vi "Page_Info_Read.vi"(6 "ctlReferences":T1, 8 "error in (no error)":errorcluster, 11 "AB_Deploy_EXE in":refnum<class "AB_Deploy_EXE.lvclass">) -> (0 "error out":errorcluster, 3 "AB_Deploy_EXE out":refnum<class "AB_Deploy_EXE.lvclass">)   [LabVIEW 2020, in "AB_Deploy_EXE.lvclass"]
uses:
  <vilib>/AppBuilder/AB_Classes/DeployableEXE/AB_Deploy_EXE.lvclass
  e:/builds/penguin/labview/branches/2020/dev/dist/vi.lib/AppBuilder/AB_Classes/Build/AB_Build.lvclass
  e:/builds/penguin/labview/branches/2020/dev/dist/vi.lib/AppBuilder/AB_Classes/TargetFile/AB_Targetfile.lvclass
  <resource>/Framework/Providers/Builds/AppBuilder/AB_UI_Page_Info_References.ctl
  <vilib>/AppBuilder/AB_Classes/DeployableEXE/AB_Deploy_EXE.lvclass/AB_Deploy_EXE.ctl
  <vilib>/AppBuilder/AB_Classes/Destination/AB_Destination.lvclass
  <vilib>/AppBuilder/AB_Classes/Build/AB_Build.lvclass
  <vilib>/AppBuilder/AB_Classes/TargetFile/AB_Targetfile.lvclass
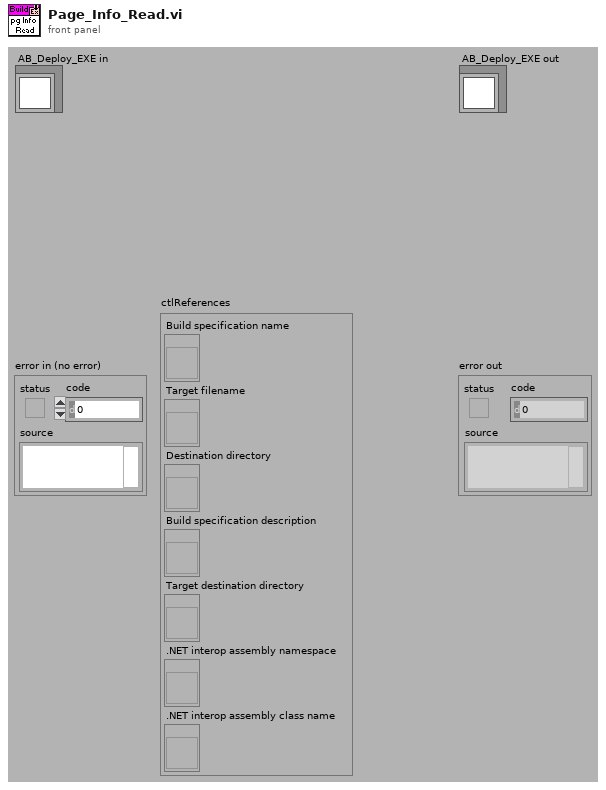
[diagram p1: front panel]
types:
  T1 = typedef "AB_UI_Page_Info_References.ctl" = cluster{"Build specification name":refnum<vi>, "Target filename":refnum<vi>, "Destination directory":refnum<vi>, "Build specification description":refnum<vi>, "Target destination directory":refnum<vi>, ".NET interop assembly namespace":refnum<vi>, ".NET interop assembly class name":refnum<vi>}
  T2 = typedef "AB_Build.ctl" = cluster{"buildSpecName":string, "buildSpecDescription":string, "destinations":refnum<class "AB_Destination.lvclass">[], "exclusionOption":T3, "defaultLanguage":string, "supportedLanguages":string[], "excludedDirectories":path[], "buildContext":refnum<vi>, "buildObject":T4, "preview":bool, "programatic":bool, "progressBarEvents":T5, "userLog_Path":path, "preActionID":string, "preAction_Path":path, "postActionID":string, "postAction_Path":path, "eng_checkForBrokenVIs?":bool, "eng_verboseLinkerErrors?":bool, "localDest_Path":path, "targetDest_Path":path, "removeVIObject":u16, "cache":refnum<class "PreviewCache.lvclass">, "use cache":bool, "previewCache_ID":string, "buildCache_ID":string, "eng_TempLocalDest_Path":path, "eng_collectDependencies?":bool, "versionInfo":cluster{"buildVersion":cluster{"major":u16, "minor":u16, "patch":u16, "build":u16}, "autoIncrement":bool}, "eng_enableVIChecksums":bool}
  T3 = typedef "AB_Exclusion_Option.ctl" = cluster{"typedefs":bool, "polymorphicVIs":bool, "unusedLibraryItems":bool, "modifyLibraryFile":bool, "edit-timeDependencies":bool, "inlineVIs":bool, "dependent PPLs":bool, "dependent DLLs":bool}
  T4 = typedef "ItemRef.ctl" = u64
  T5 = typedef "provcom_ProgressBar_Events.ctl" = cluster{"newJob":refnum<user-event>, "newItem":refnum<user-event>, "errorMsg":T6, "cancel":refnum<user-event>}
  T6 = typedef "mxLvBuildError.ctl" = refnum<user-event>
  T7 = typedef "AB_Targetfile.ctl" = cluster{"targetfileName":string, "targetfileGUID":string, "enableDebugging":bool, "versionInfo":cluster{"productName":string, "legalCopyright":string, "companyName":string, "internalName":string, "fileDescription":string}, "eng_consolidatedTypeInfo":string, "fastFileFormat":bool, "eng_LEIFBuildData":u32, "versionIndependent":bool}
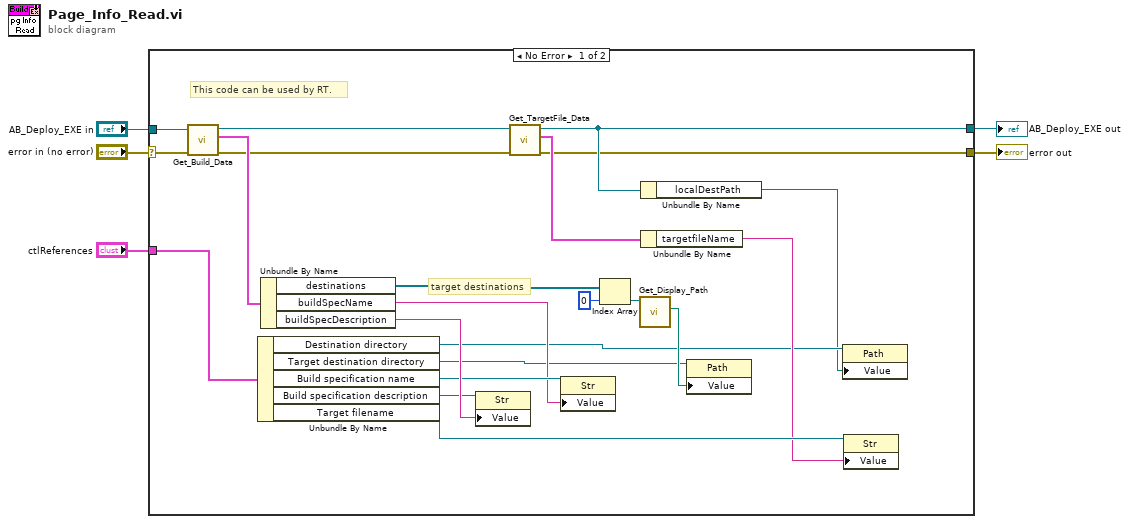
[diagram p0: block diagram]
diagram:
  n1 = case shown="No Error" "error in (no error)" {
    selector: "error in (no error)" -> [w26 w29]
    tunnel: [w6 w29] -> w4
    tunnel: "AB_Deploy_EXE in" -> [w27 w28]
    tunnel: "ctlReferences" -> [w24 _]
    tunnel: [w7 w28] -> w1
    frame No Error {
      # "This code can be used by RT."
      # "target destinations"
      n2 = call <vilib>:"Get_Build_Data.vi"("error in (no error)"=w26, "Class in"=w27) -> ("error out"=w13:errorcluster, "data"=w25:T2, "Class out"=w14:refnum<class "AB_Deploy_EXE.lvclass">)  [unwired: 7 in]
      n3 = Unbundle By Name(w24) -> ("Destination directory"=w9:refnum<vi>, "Target destination directory"=w15:refnum<vi>, "Build specification name"=w19:refnum<vi>, "Build specification description"=w20:refnum<vi>, "Target filename"=w11:refnum<vi>)
      n4 = Unbundle By Name(w25) -> ("destinations"=w17:refnum<class "AB_Destination.lvclass">[], "buildSpecName"=w18:string, "buildSpecDescription"=w21:string)
      n5 = property class="Str"(reference=w20, "Value"=w21) -> ()  [unwired: 1 in, 2 out]
      n6 = call <vilib>:"Get_TargetFile_Data.vi"("error in (no error)"=w13, "AB_Targetfile in"=w14) -> ("error out"=w6:errorcluster, "data"=w12:T7, "AB_Targetfile out"=w7:refnum<class "AB_Deploy_EXE.lvclass">)  [unwired: 7 in]
      n7 = property class="Str"(reference=w19, "Value"=w18) -> ()  [unwired: 1 in, 2 out]
      n8 = Index Array(array=w17, index=0) -> (element=w16:refnum<class "AB_Destination.lvclass">)
      n9 = call-dynamic "Get_Display_Path.vi"("AB_Destination in"=w16) -> ("displayPath"=w23:path)  [unwired: 8 in, 2 out]
      n10 = Unbundle By Name(w7) -> ("localDestPath"=w8:path)
      n11 = Unbundle By Name(w12) -> ("targetfileName"=w10:string)
      n12 = property class="Path"(reference=w15, "Value"=w23) -> ()  [unwired: 1 in, 2 out]
      n13 = property class="Path"(reference=w9, "Value"=w8) -> ()  [unwired: 1 in, 2 out]
      n14 = property class="Str"(reference=w11, "Value"=w10) -> ()  [unwired: 1 in, 2 out]
    }
    frame Error {
    }
  }
  "error out" <- w4
  "AB_Deploy_EXE out" <- w1
